vi "GetParam.vi"(8 "error in (no error)":errorcluster caption="entrée d'erreur (pas d'erreur)", 11 "Nan_euclidean_distances.lvclass":refnum<class "Nan_euclidean_distances.lvclass">) -> (0 "error out":errorcluster caption="sortie d'erreur", 2 "nan_euclidean_distances":T1={"squared"=FALSE, "missing_values"="nan", "copy"=TRUE}, 3 "Nan_euclidean_distances.lvclass":refnum<class "Nan_euclidean_distances.lvclass">)   [LabVIEW 2020, in "Nan_euclidean_distances.lvclass"]
doc: "Get Parameters"
uses:
  Nan_euclidean_distances.lvclass
  Nan_euclidean_distances.lvclass/Nan_euclidean_distances.ctl
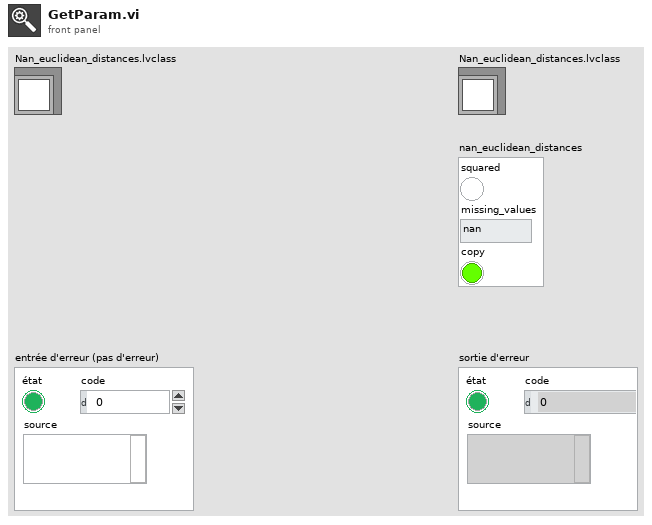
[diagram p1: front panel]
types:
  T1 = cluster{"squared":bool, "missing_values":string, "copy":bool}
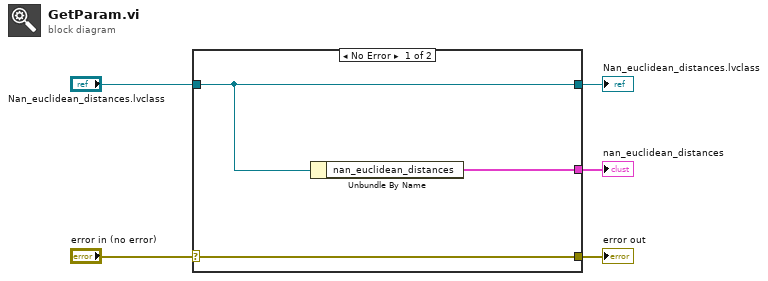
[diagram p0: block diagram]
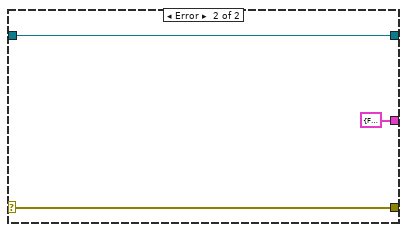
[diagram p2: hidden frame]
diagram:
  n1 = case shown="No Error" "error in (no error)" {
    selector: "error in (no error)" -> [w8 w10]
    tunnel: [w8 w10] -> w4
    tunnel: [w7 w11] -> w2
    tunnel: "Nan_euclidean_distances.lvclass" -> [w7 w11]
    tunnel: [w6 T1 {"squared"=FALSE, "missing_values"="", "copy"=FALSE} ("nan_euclidean_distances")] -> w1
    frame No Error {
      n2 = Unbundle By Name(w7) -> ("nan_euclidean_distances"=w6:T1)
    }
    frame Error {
    }
  }
  "error out" <- w4
  "Nan_euclidean_distances.lvclass" <- w2
  "nan_euclidean_distances" <- w1
